vi "TagBus_Read Table to Cluster (DVR).vi"(7 "Clust Refnum":refnum<vi>, 10 "Index Array":i32[](array[numeric]), 11 "TagBus DVR":refnum<data-value>) -> (3 "TagBus DVR out":refnum<data-value>)   [LabVIEW 2015, in "TagBus.lvclass"]
uses:
  TagBus.lvclass
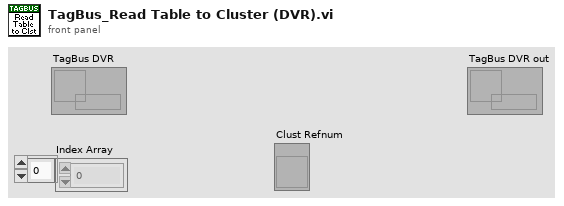
[diagram p1: front panel]
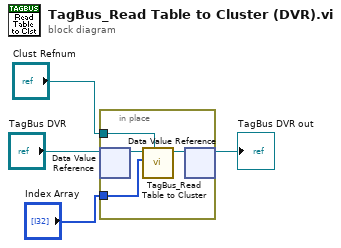
[diagram p0: block diagram]
diagram:
  n1 = in-place {
    in-place-border: "Index Array" -> [w6]
    in-place-border: "Clust Refnum" -> [w5]
    n2 = in-place-dvr #1("TagBus DVR") -> (w8:refnum<class "TagBus.lvclass">)  [unwired: 1 out]
    n3 = call "TagBus_Read Table to Cluster.vi"("Clust Refnum"=w5, "Index Array"=w6, "TagBus"=w8) -> ("TagBus out"=w7:refnum<class "TagBus.lvclass">)  [unwired: 8 in]
    n4 = in-place-dvr #1(w7) -> (→"TagBus DVR out":refnum<data-value>)  [unwired: 1 out]
  }
